vi "set_volume_leds_avg.vi"(8 "error in (no error)":errorcluster, 9 "Array":dbl[](array[numeric]), 10 "Numeric":i32=10, 11 "Refnum in":refnum<k21>) -> (0 "error out":errorcluster, 3 "Refnum out":refnum<k21>)   [LabVIEW 2022 SP3]
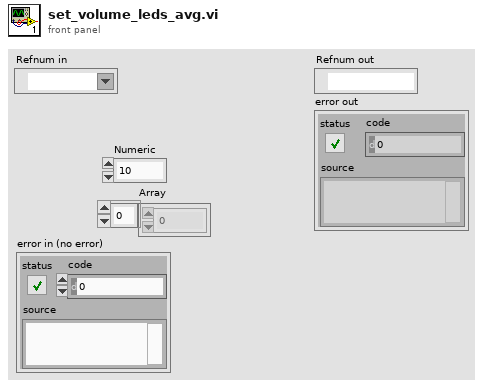
[diagram p1: front panel]
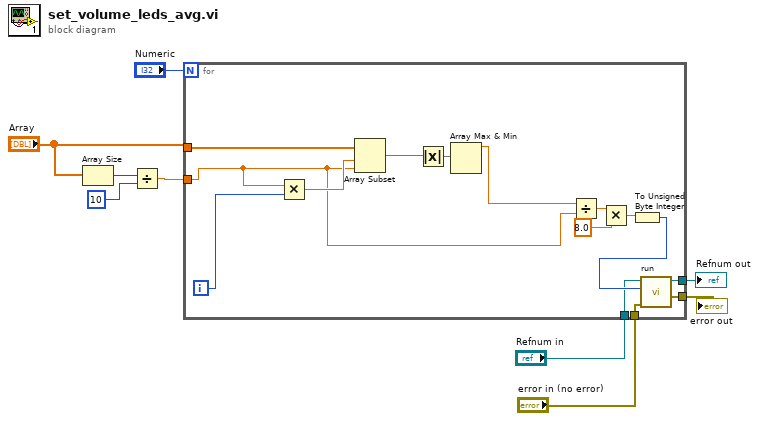
[diagram p0: block diagram]
diagram:
  n1 = Array Size(array="Array") -> (size(s)=w7:i32)
  n2 = Divide(x=w7, y=10) -> (x/y=w5:dbl)
  n3 = for {
    N: "Numeric" -> [_]
    tunnel: "Array" -> [w24]
    tunnel: w5 -> [w13]
    tunnel: "Refnum in" -> [w17]
    tunnel: "error in (no error)" -> [w16]
    tunnel: [w15] -> w2
    tunnel: [w14] -> w1
    i -> [w23]
    n4 = Multiply(x=w13, y=w23) -> (x*y=w22:dbl)
    n5 = Array Subset(array=w24, index=w22, length=w13) -> (w12:dbl[])
    n6 = Absolute Value(x=w12) -> (abs(x)=w11:dbl[])
    n7 = Array Max & Min(array=w11) -> (max value=w10:dbl)  [unwired: 3 out]
    n8 = Divide(x=w10, y=w13) -> (x/y=w21:dbl)
    n9 = Multiply(x=w21, y=8.0) -> (x*y=w19:dbl)
    n10 = To Unsigned Byte Integer(number=w19) -> (unsigned 8bit integer=w18:u8)
    n11 = call "run.vi"("error in (no error)"=w16, "volume"=w18, "Refnum in"=w17) -> ("error out"=w14:errorcluster, "Refnum out"=w15:refnum<k21>)  [unwired: 7 in]
  }
  "Refnum out" <- w2
  "error out" <- w1
